vi "FT_Read_String_Data.vi"(0 "Handle":u32, 1 "Bytes To Read":u32) -> (2 "FT_Status":u32, 3 "Read Data":string, 4 "Bytes Read":u32, 5 "Handle":u32)   [LabVIEW 2011]
uses:
  FTD2XX.dll
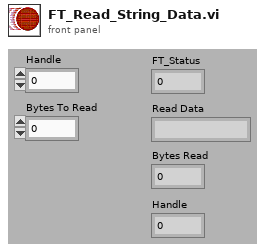
[diagram p1: front panel]
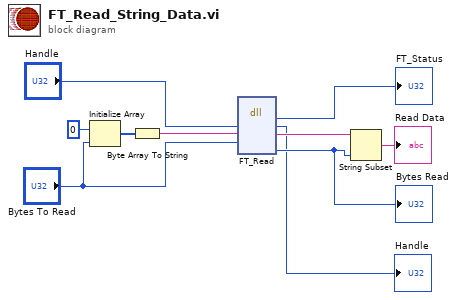
[diagram p0: block diagram]
diagram:
  n1 = Initialize Array(u8 0, "Bytes To Read") -> (w7:u8[])
  n2 = Byte Array To String(unsigned byte array=w7) -> (string=w6:string)
  n3 = dll-call lib="C:/Work/Labview/#Avesta/D2XX_Functions_7.0/FTD2XX.dll" fn="FT_Read"("Handle"="Handle", "Buffer"=w6, "BytesToRead"="Bytes To Read") -> ("FT_Status"=→"FT_Status":u32, "Handle"=→"Handle":u32, "Buffer"=w3:string, "BytesReturned"=w2:u32)  [unwired: 4 in, 3 out]
  "Bytes Read" <- w2
  n4 = String Subset(string=w3, length (rest)=w2) -> (substring=→"Read Data":string)  [unwired: 1 out]
